vi "查询启动项.vi"(8 "error in (no error)":errorcluster caption="错误输入（无错误）") -> (0 "error out":errorcluster caption="错误输出", 3 "包含启动项":bool)   [LabVIEW 2016]
uses:
  <vilib>/registry/registry.llb/Registry RtKey.ctl
  <vilib>/registry/registry.llb/Registry SAM.ctl
panel:
  out "values":string[](array[string]) caption="值"
  out "字符串":string
  out "String/Binary data":string[](array[string]) caption="字符串/二进制数据"
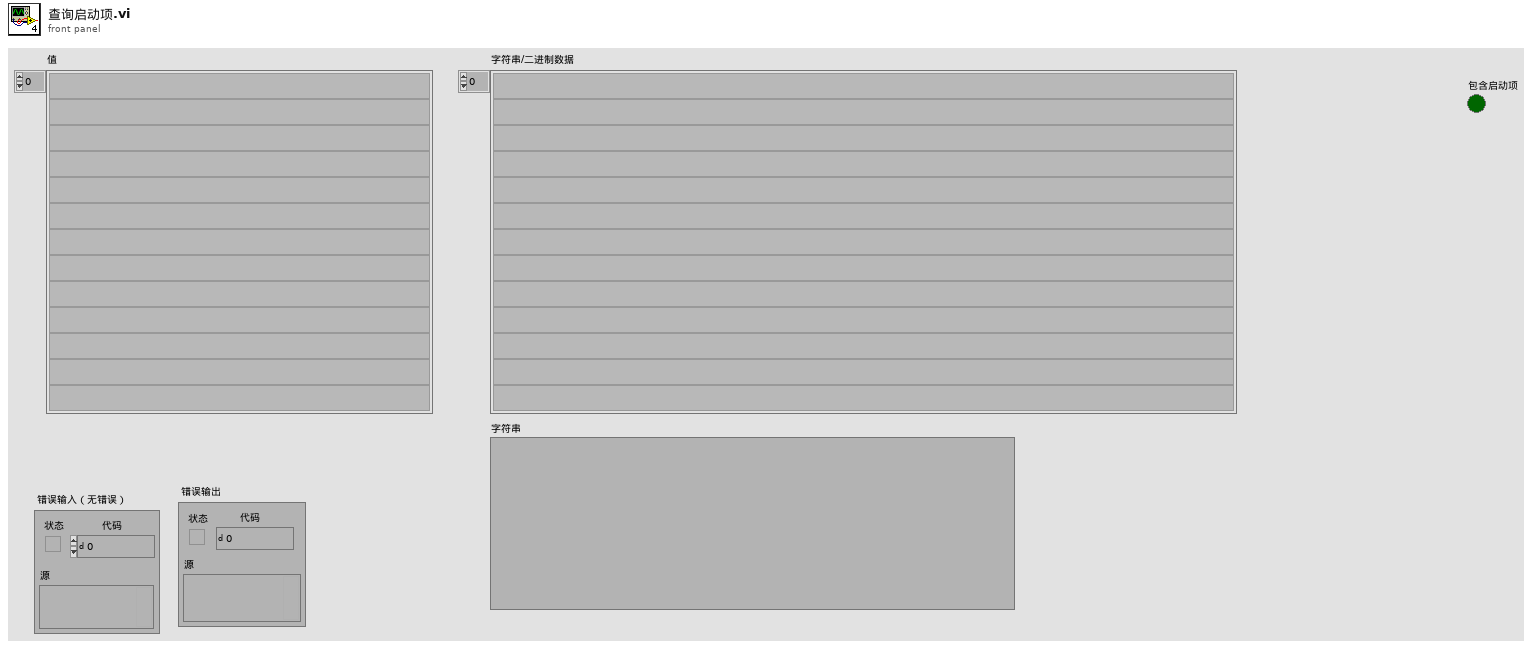
[diagram p1: front panel]
types:
  T1 = typedef "Registry SAM.ctl" = enum32{"KEY_QUERY_VALUE", "KEY_SET_VALUE", "KEY_CREATE_SUB_KEY", "KEY_ENUMERATE_SUB_KEYS", "KEY_NOTIFY", "KEY_CREATE_LINK", "KEY_READ", "KEY_WRITE", "KEY_ALL_ACCESS", "KEY_READ | KEY_WRITE"}
  T2 = typedef "Registry RtKey.ctl" = enum32{"HKEY_CLASSES_ROOT", "HKEY_CURRENT_USER", "HKEY_LOCAL_MACHINE", "HKEY_USERS", "HKEY_PERFORMANCE_DATA", "HKEY_CURRENT_CONFIG", "HKEY_DYN_DATA"}
  T3 = typedef "Registry refnum.ctl" = refnum<k1>
  T4 = cluster{"numValues":i32, "maxValueNameLen":i32, "maxValueDataLen":i32}
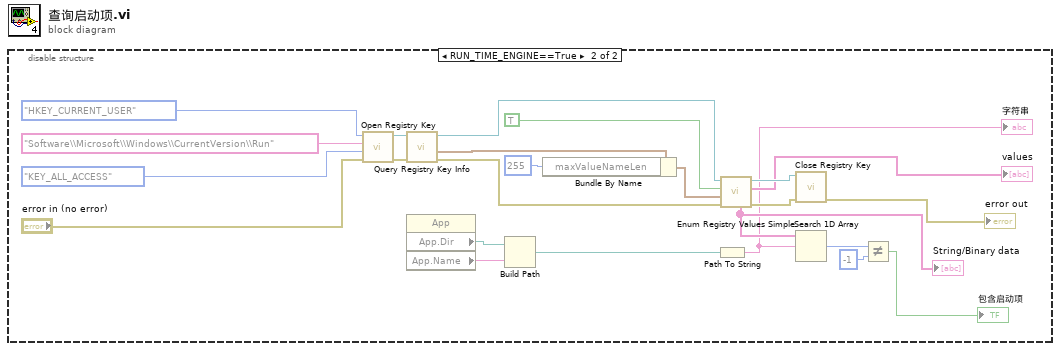
[diagram p0: block diagram]
diagram:
  n1 = disable-structure shown="RUN_TIME_ENGINE==True" {
    frame condition #0 (active) {
    }
    frame condition #1 {
      n2 = call <vilib>:"Open Registry Key.vi"("error in (no error)"="error in (no error)", "security access mask (KEY_READ | KEY_WRITE)"=Registry_SAM."KEY_ALL_ACCESS", "subkey"="Software\\Microsoft\\Windows\\CurrentVersion\\Run", "root key (HKEY_LOCAL_MACHINE)"=Registry_RtKey."HKEY_CURRENT_USER") -> ("error out"=w21:errorcluster, "refnum out"=w22:T3)  [unwired: 6 in]
      n3 = call <vilib>:"Query Registry Key Info.vi"("error in (no error)"=w21, "refnum"=w22) -> ("error out"=w18:errorcluster, "value info"=w19:T4, "refnum out"=w20:T3)  [unwired: 5 in, 2 out]
      n4 = property class="App"() -> ("App.Dir"=w6:path, "App.Name"=w5:string)  [unwired: 2 in, 2 out]
      n5 = Build Path(base path=w6, name or relative path=w5) -> (appended path=w4:path)
      n6 = Bundle By Name(cluster=w19, "maxValueNameLen"=255) -> (w9:T4)
      n7 = Path To String(path=w4) -> (string=w1:string)
      "字符串" <- w1
      n8 = call <vilib>:"Enum Registry Values Simple.vi"("error in (no error)"=w18, "value info"=w9, "retrieve data? (F)"=TRUE, "refnum"=w20) -> ("error out"=w16:errorcluster, "values"=→"values":string[], "refnum out"=w17:T3, "String/Binary data"=w3:string[])  [unwired: 2 in, 2 out]
      "String/Binary data" <- w3
      n9 = call <vilib>:"Close Registry Key.vi"("error in (no error)"=w16, "refnum"=w17) -> ("error out"=→"error out":errorcluster)  [unwired: 5 in]
      n10 = Search 1D Array(1D array=w3, element=w1) -> (index of element=w15:i32)  [unwired: 1 in]
      n11 = Not Equal?(x=w15, y=-1) -> (x != y?=→"包含启动项":bool)
    }
  }
